vi "Update Disc Count.vi"(5 "Reset":bool, 6 "Manual Subtract":bool, 7 "Manual Add":bool, 8 "Disc IR Hopper":bool, 9 "Disc IR Shooter":bool, 10 "Flipper":bool, 11 "Disc Mode":enum16{"Drive", "Load", "Shoot", "Feed"}(ring)) -> (3 "Disc Count out":dbl)   [LabVIEW 2013]
uses:
  Robot Global Data.vi
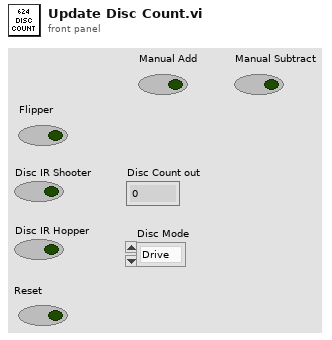
[diagram p1: front panel]
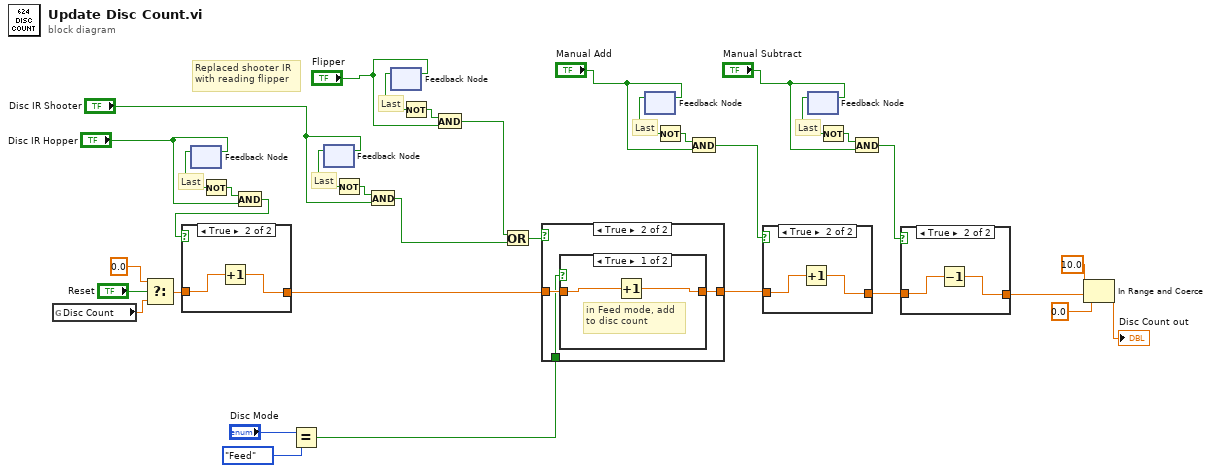
[diagram p0: block diagram]
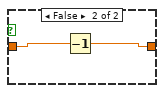
[diagram p5: hidden frame]
diagram:
  # "Last"
  # "Last"
  # "Replaced shooter IR\nwith reading flipper"
  # "Last"
  # "Last"
  # "Last"
  n1 = global read "Robot Global Data.vi" "Disc Count"() -> (w19:dbl)
  n2 = Select(t=0.0, s="Reset", f=w19) -> (s? t:f=w18:dbl)
  n3 = feedback #1() -> (w28:bool)  [unwired: 1 in]
  n4 = feedback-in #1("Disc IR Hopper") -> ()
  n5 = Not(x=w28) -> (.not. x?=w29:bool)
  n6 = And(x=w29, y="Disc IR Hopper") -> (x .and. y?=w31:bool)
  n7 = case shown="True" w31 {
    tunnel: w18 -> [w36 w38]
    tunnel: [w36 w37] -> w35
    frame False {
    }
    frame True {
      n8 = Increment(x=w38) -> (x+1=w37:dbl)
    }
  }
  n9 = Equal?(x="Disc Mode", y=enum16{"Drive", "Load", "Shoot", "Feed"}."Feed") -> (x = y?=w25:bool)
  n10 = feedback #2() -> (w33:bool)  [unwired: 1 in]
  n11 = feedback-in #2("Disc IR Shooter") -> ()
  n12 = Not(x=w33) -> (.not. x?=w32:bool)
  n13 = And(x=w32, y="Disc IR Shooter") -> (x .and. y?=w13:bool)
  n14 = feedback #3() -> (w16:bool)  [unwired: 1 in]
  n15 = feedback-in #3("Flipper") -> ()
  n16 = Not(x=w16) -> (.not. x?=w17:bool)
  n17 = And(x=w17, y="Flipper") -> (x .and. y?=w12:bool)
  n18 = Or(x=w12, y=w13) -> (x .or. y?=w14:bool)
  n19 = case shown="True" w14 {
    tunnel: w35 -> [w39 w42]
    tunnel: [w39 w41] -> w11
    tunnel: w25 -> [_ w40]
    frame False {
    }
    frame True {
      n20 = case shown="True" w40 {
        tunnel: w42 -> [w44 w46]
        tunnel: [w43 w45] -> w41
        frame True {
          # "in Feed mode, add\nto disc count"
          n21 = Increment(x=w44) -> (x+1=w43:dbl)
        }
        frame False {
          n22 = Decrement(x=w46) -> (x-1=w45:dbl)
        }
      }
    }
  }
  n23 = feedback #4() -> (w8:bool)  [unwired: 1 in]
  n24 = feedback-in #4("Manual Add") -> ()
  n25 = Not(x=w8) -> (.not. x?=w7:bool)
  n26 = And(x=w7, y="Manual Add") -> (x .and. y?=w2:bool)
  n27 = case shown="True" w2 {
    tunnel: w11 -> [w47 w49]
    tunnel: [w47 w48] -> w10
    frame False {
    }
    frame True {
      n28 = Increment(x=w49) -> (x+1=w48:dbl)
    }
  }
  n29 = feedback #5() -> (w5:bool)  [unwired: 1 in]
  n30 = feedback-in #5("Manual Subtract") -> ()
  n31 = Not(x=w5) -> (.not. x?=w6:bool)
  n32 = And(x=w6, y="Manual Subtract") -> (x .and. y?=w1:bool)
  n33 = case shown="True" w1 {
    tunnel: w10 -> [w50 w52]
    tunnel: [w50 w51] -> w9
    frame False {
    }
    frame True {
      n34 = Decrement(x=w52) -> (x-1=w51:dbl)
    }
  }
  n35 = In Range and Coerce(upper limit=10.0, x=w9, lower limit=0.0) -> (coerced(x)=→"Disc Count out":dbl)  [unwired: 1 out]
